vi "Main_UI.vi"() -> ()   [LabVIEW 2020, in "Airplane CLD1.lvlib"]
doc: "This is an Airplane Lavatory. This shows if the front and rear are occupied. The Steward's area controls the signals and Alarm."
uses:
  Airplane CLD1.lvlib
  Input_Cluster.ctl
panel:
  in  "Stop":bool
  out "Error out":errorcluster
  in  "Error in":errorcluster
  in  "Alarm Timer Limit":dbl=10.0
  out "Alarm Timer D":dbl
  out "Alarm Timer C":dbl
  out "Alarm Timer B":dbl
  out "Alarm Timer A":dbl
  out "Lavatory":string
  in  "Alarm Acknowledge":bool
  out "Alarm":bool
  in  "Seatbelt Sign ON":bool
  out "Lavatories \nOccupied\nRear":bool
  out "Lavatories \nOccupied\nFront":bool
  in  "Lavatory D Occupied":bool
  in  "Lavatory C Occupied":bool
  in  "Lavatory B Occupied":bool
  in  "Lavatory A Occupied":bool
  out "Return to Seat B":bool
  out "Occupied B":bool
  out "Return to Seat A":bool
  out "Occupied A":bool
  out "Return to Seat D":bool
  out "Occupied D":bool
  out "Return to Seat C":bool
  out "Occupied C":bool
  # "AIRPLANE LAVATORY SIGNS"
  # "FRONT"
  # "REAR"
  # "LAVATORY A"
  # "LAVATORY C"
  # "STEWARDS'S AREA"
  # "LAVATORY B"
  # "LAVATORY D"
  # "SIMULATION CONTROLS & INDICATORS"
  # "secs"
  # "secs"
  # "secs"
  # "secs"
  # "secs"
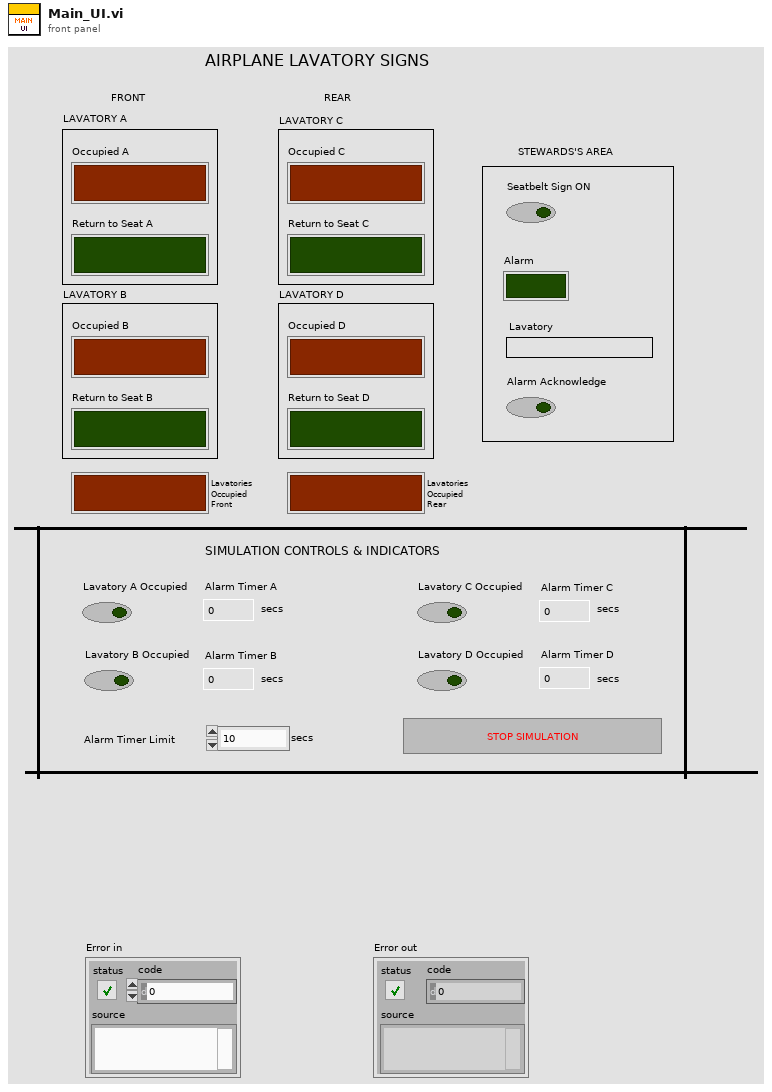
[diagram p1: front panel]
types:
  T1 = typedef "Airplane CLD1.lvlib/Input_Cluster.ctl" = cluster{"Occupied A":bool, "Occupied B":bool, "Occupied C ":bool, "Occupied D":bool, "Lavatories \nOccupied\nFront":bool, "Lavatories \nOccupied\nRear":bool, "Return":bool, "A Initial":dbl, "B Initial":dbl, "C Initial":dbl, "D Initial":dbl, "Alarm Timer A":dbl, "Alarm Timer B":dbl, "Alarm Timer C":dbl, "Alarm Timer D":dbl, "Alarm Timer Limit":dbl, "Lavatory":string, "Alarm":bool, "Alarm Acknowledge":bool}
  T2 = enum16{"Create Queue", "Enqueue element", "Enqueue N elements", "Dequeue", "Enstack 1 element", "Flush Queue", "Close Queue"}
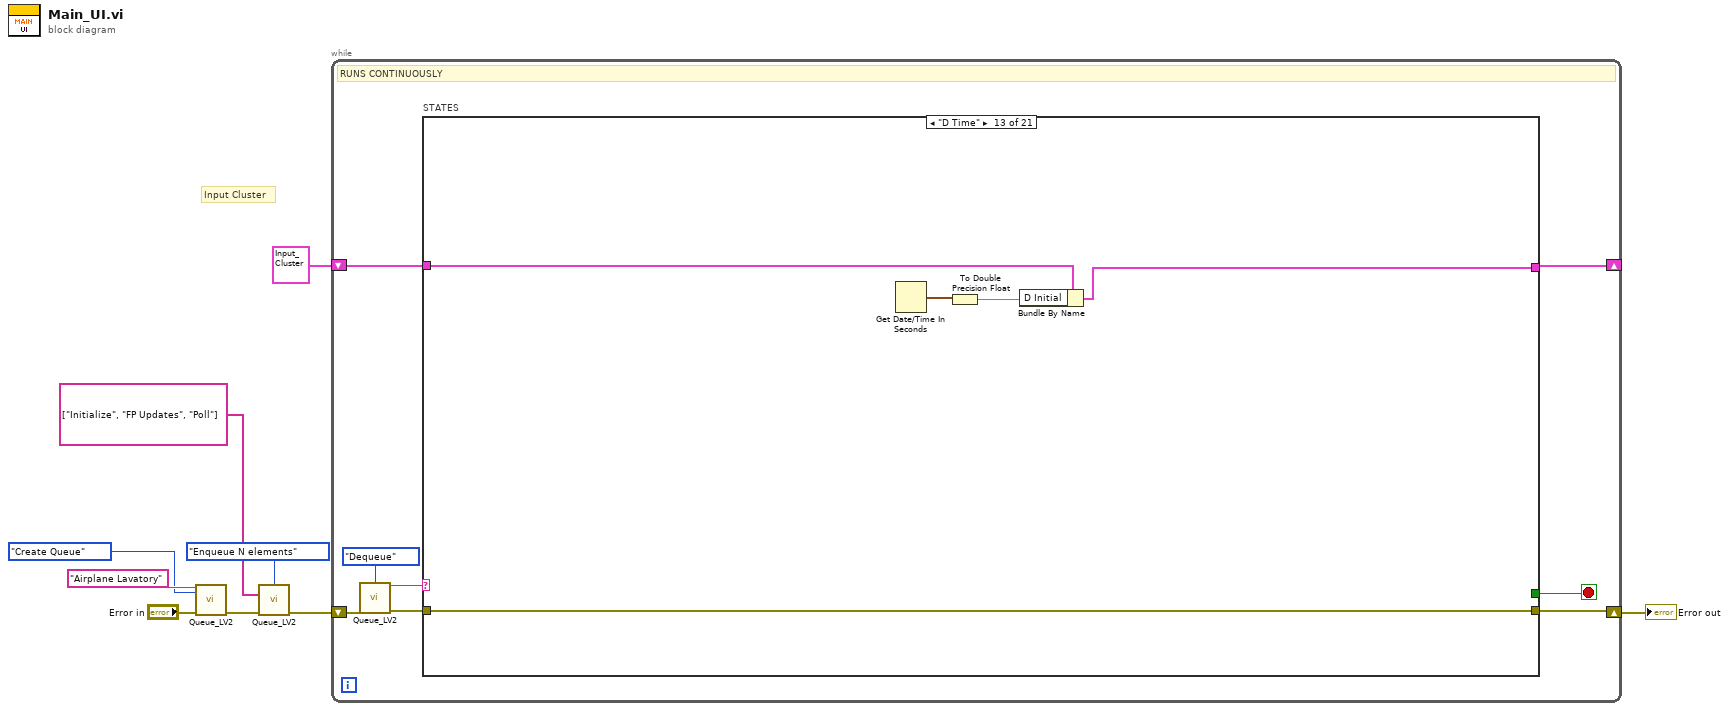
[diagram p0: block diagram]
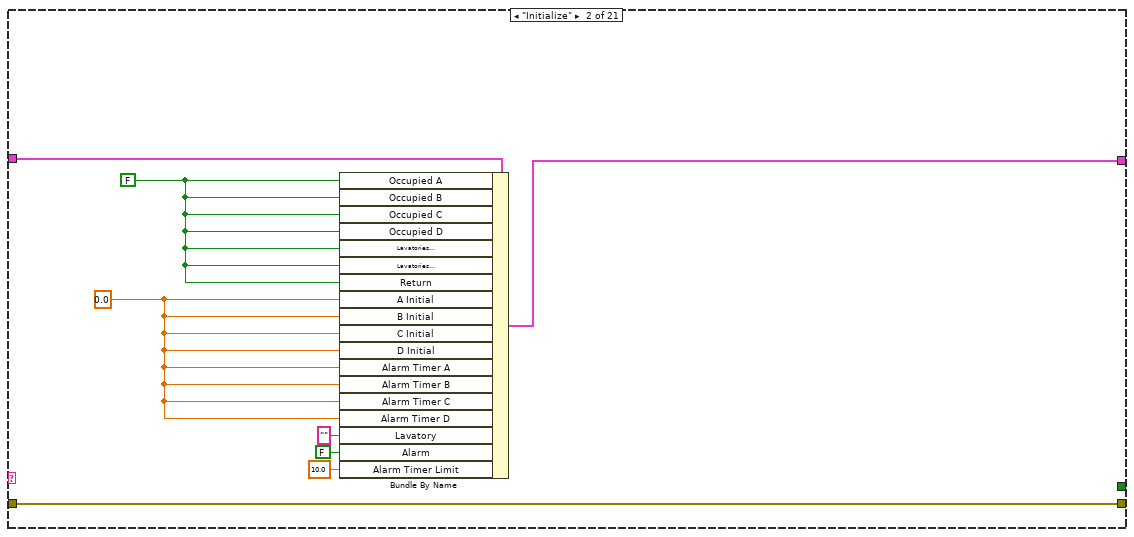
[diagram p3: hidden frame]
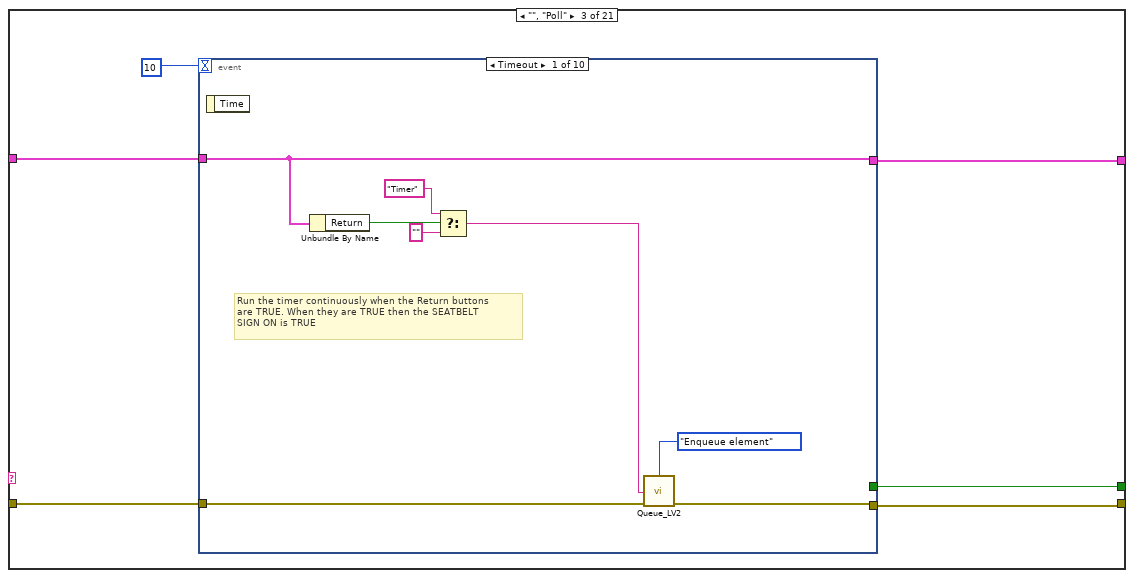
[diagram p4: hidden frame]
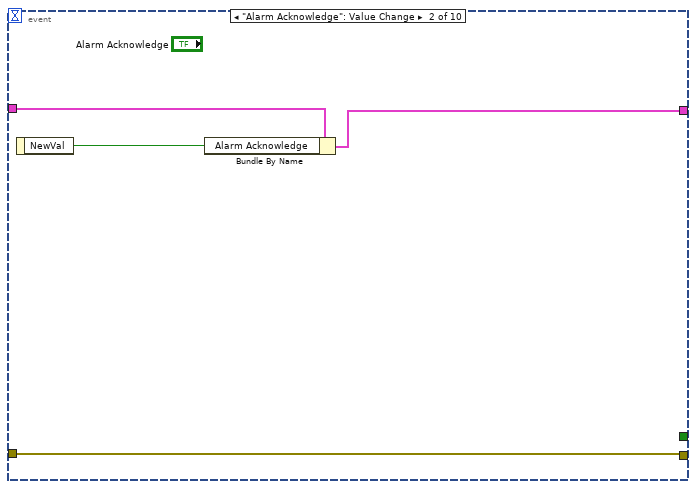
[diagram p5: hidden frame]
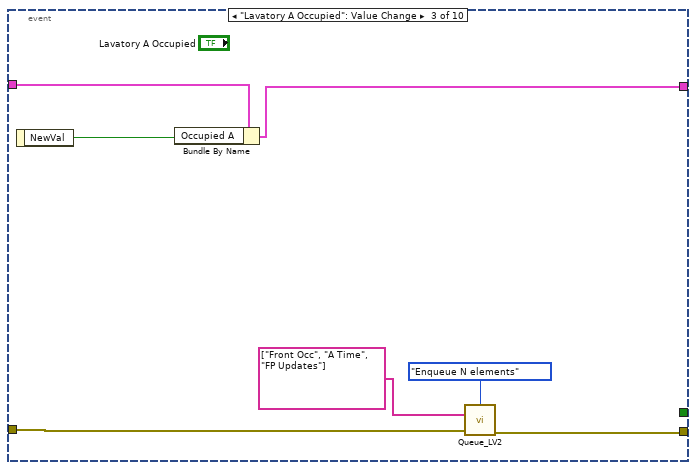
[diagram p6: hidden frame]
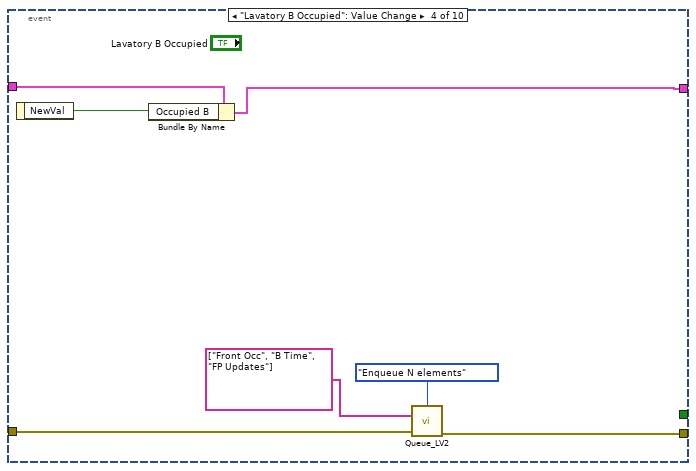
[diagram p7: hidden frame]
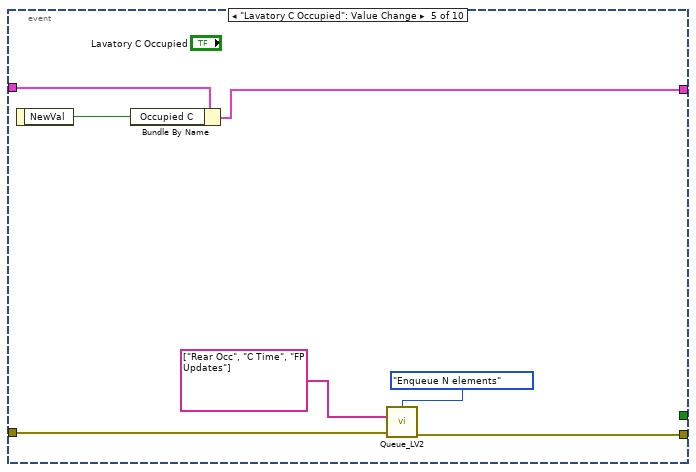
[diagram p8: hidden frame]
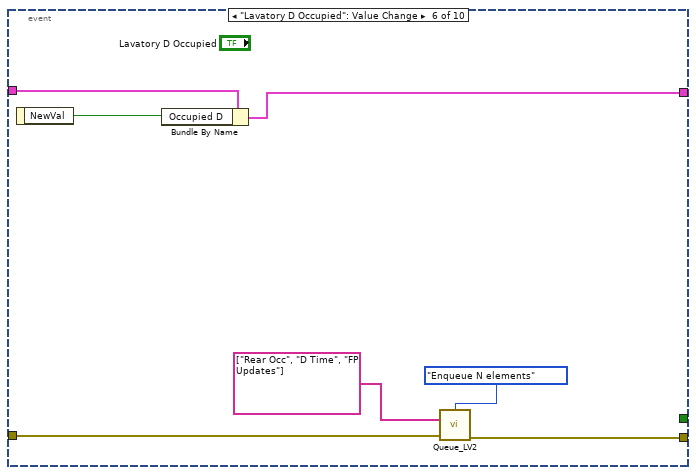
[diagram p9: hidden frame]
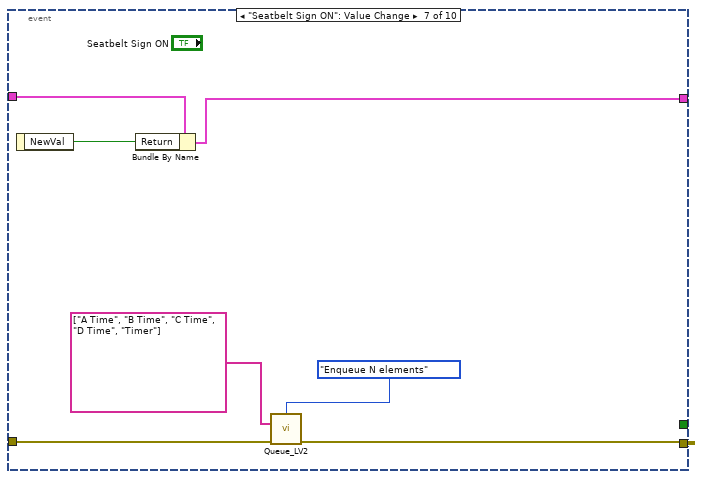
[diagram p10: hidden frame]
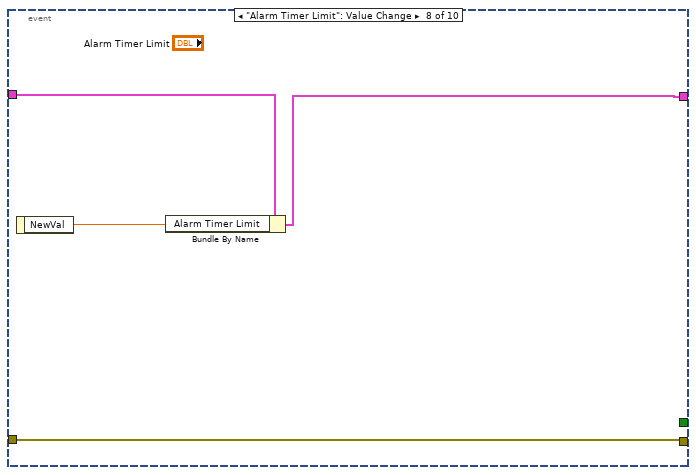
[diagram p11: hidden frame]
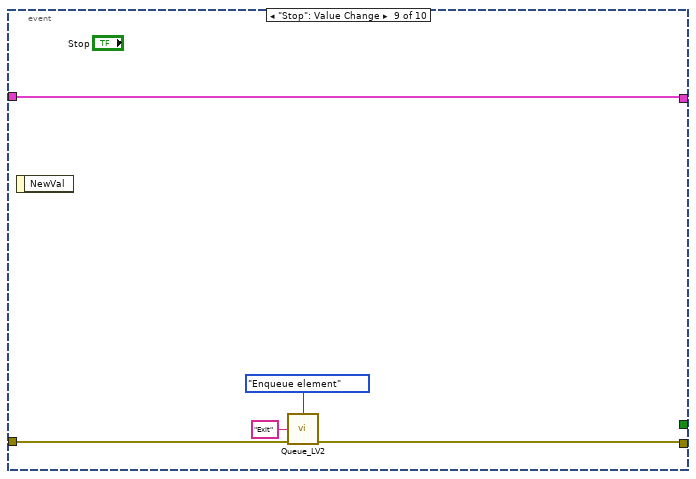
[diagram p12: hidden frame]
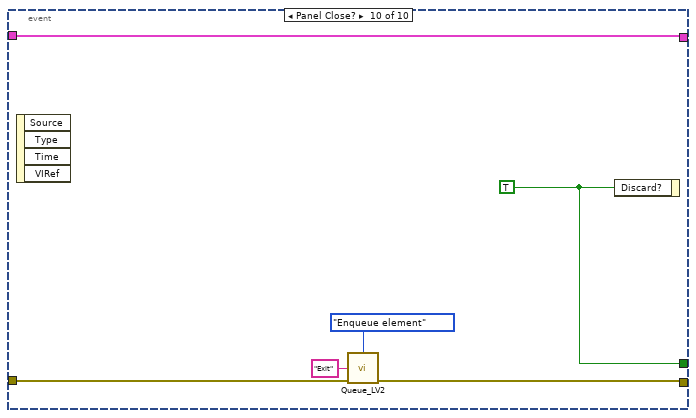
[diagram p13: hidden frame]
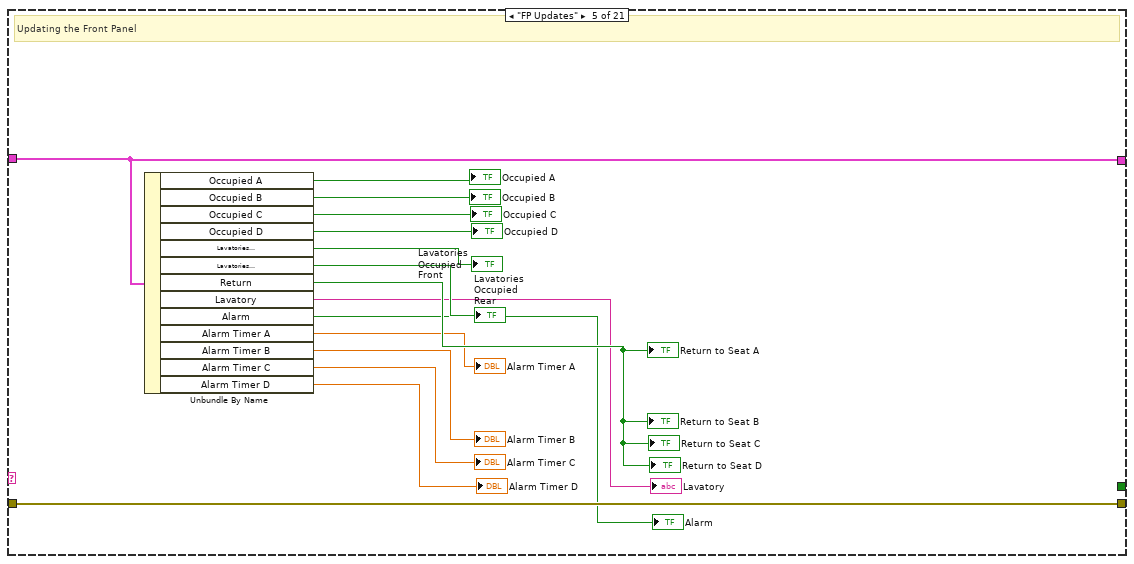
[diagram p15: hidden frame]
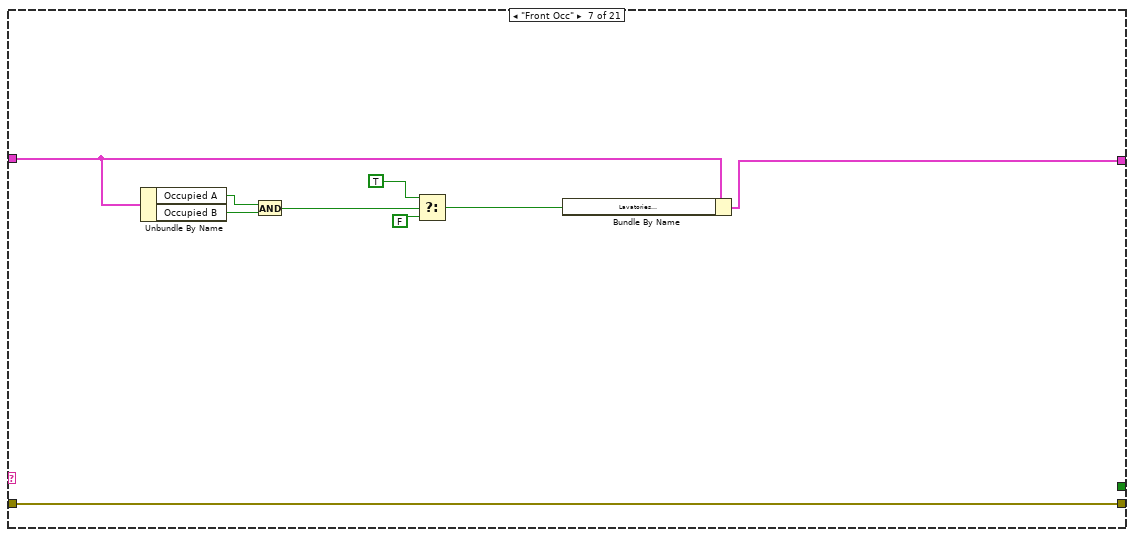
[diagram p17: hidden frame]
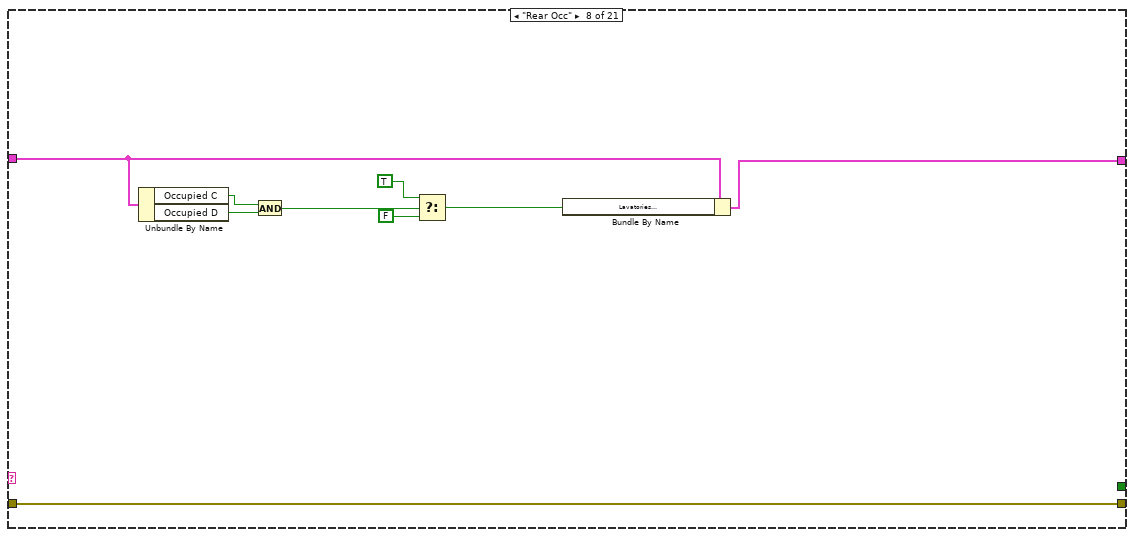
[diagram p18: hidden frame]
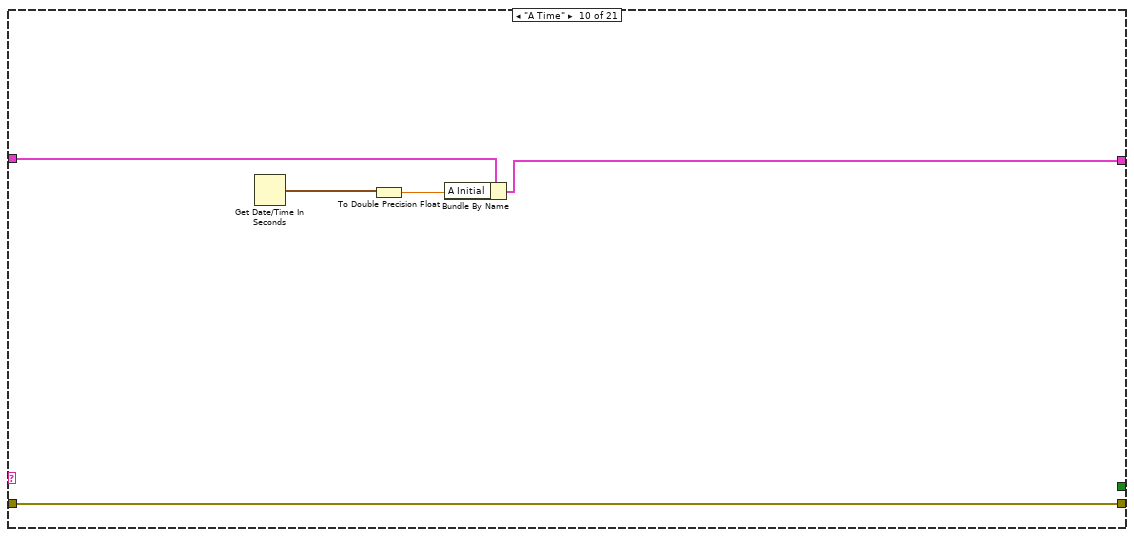
[diagram p20: hidden frame]
diagram:
  # "Input Cluster"
  n1 = call "Queue_LV2.vi"("name"="Airplane Lavatory", "Queue Operations"=T2."Create Queue", "error in"="Error in") -> ("error out"=w7:errorcluster)  [unwired: 11 in, 1 out]
  n2 = call "Queue_LV2.vi"("Queue Operations"=T2."Enqueue N elements", "States[]"=string[] ["Initialize", "FP Updates", "Poll"], "error in"=w7) -> ("error out"=w5:errorcluster)  [unwired: 11 in, 1 out]
  n3 = while {
    shift-right: [w13] -> w2
    shift-left: w5 -> [w17]
    shift-right: [w10] -> _
    shift-left: T1 {"Occupied A"=FALSE, "Occupied B"=FALSE, "Occupied C "=FALSE, "Occupied D"=FALSE, "Lavatories \nOccupied\nFront"=FALSE, "Lavatories \nOccupied\nRear"=FALSE, "Return"=FALSE, "A Initial"=0.0, "B Initial"=0.0, "C Initial"=0.0, "D Initial"=0.0, "Alarm Timer A"=0.0, "Alarm Timer B"=0.0, "Alarm Timer C"=0.0, "Alarm Timer D"=0.0, "Alarm Timer Limit"=0.0, "Lavatory"="", "Alarm"=FALSE, "Alarm Acknowledge"=FALSE} -> [w11]
    stop <- w12 stop-if-true
    # "RUNS CONTINUOUSLY"
    n4 = call "Queue_LV2.vi"("Queue Operations"=T2."Dequeue", "error in"=w17) -> ("DQ State"=w15:string, "error out"=w14:errorcluster)  [unwired: 12 in]
    n5 = case "STATES" shown="\"D Time\"" w15 {
      selector: w15 -> [_ _ _ _ _ _ _ _ _ _ _ _ _ _ _ _ _ _ w249 _ _]
      tunnel: w14 -> [w19 w27 w30 w96 w107 w113 w123 w132 w133 w135 w140 w145 w150 w155 w158 w190 w204 w245 w250 w251 w258]
      tunnel: [w19 w27 w29 w96 w107 w113 w123 w132 w133 w135 w140 w145 w150 w155 w159 w190 w200 w245 w250 w251 w254] -> w13
      tunnel: [_ _ w28 _ _ _ _ _ _ _ _ _ _ _ _ _ _ _ w248 _ TRUE ("true")] -> w12
      tunnel: w11 -> [w18 w26 w32 w97 w108 w114 w117 w124 w134 w139 w142 w147 w152 w156 w166 w191 w219 w246 w247 w252 w259]
      tunnel: [w18 w25 w31 w97 w108 w114 w116 w125 w134 w136 w141 w146 w151 w156 w165 w191 w217 w246 w247 w252 w259] -> w10
      frame "/****Initialize****/" {
        # "Splitter Case"
      }
      frame "Initialize" {
        w23 = 0.0
        w24 = FALSE ("Occupied A")
        n6 = Bundle By Name(cluster=w26, "Occupied A"=w24, "Occupied B"=w24, "Occupied C"=w24, "Occupied D"=w24, "Lavatories \nOccupied\nFront"=w24, "Lavatories \nOccupied\nRear"=w24, "Return"=w24, "A Initial"=w23, "B Initial"=w23, "C Initial"=w23, "D Initial"=w23, "Alarm Timer A"=w23, "Alarm Timer B"=w23, "Alarm Timer C"=w23, "Alarm Timer D"=w23, "Lavatory"="", "Alarm"=FALSE, "Alarm Timer Limit"=10.0) -> (w25:T1)
      }
      frame "", "Poll" {
        n7 = event shown="[0] Timeout" {
          selector: _ -> [_ _ _ _ _ _ _ _ _ _]
          dyn-events: _ -> [_ _ _ _ _ _ _ _ _ _]
          timeout: 10 -> [_ _ _ _ _ _ _ _ _ _]
          tunnel: w32 -> [w41 w45 w52 w59 w66 w73 w80 w84 w85 w94]
          tunnel: [w41 w44 w50 w58 w65 w72 w78 w82 w85 w94] -> w31
          tunnel: w30 -> [w35 w42 w47 w54 w61 w70 w77 w81 w89 w93]
          tunnel: [w34 w42 w46 w53 w60 w69 w76 w81 w88 w92] -> w29
          tunnel: [_ _ _ _ _ _ _ _ _ w95] -> w28
          event Timeout {
            # "Run the timer continuously when the Return buttons\nare TRUE. When they are TRUE then the SEATBELT\nSIGN ON is TRUE"
            n8 = event-data() -> ()  [unwired: 1 in, 1 out]
            n9 = Unbundle By Name(w41) -> ("Return"=w40:bool)
            n10 = Select(t="Timer", s=w40, f="") -> (s? t:f=w37:string)
            n11 = call "Queue_LV2.vi"("Queue Operations"=T2."Enqueue element", "State"=w37, "error in"=w35) -> ("error out"=w34:errorcluster)  [unwired: 11 in, 1 out]
          }
          event "Alarm Acknowledge": Value Change {
            n12 = event-data() -> ("NewVal"=w43:bool)  [unwired: 1 in]
            n13 = Bundle By Name(cluster=w45, "Alarm Acknowledge"=w43) -> (w44:T1)
          }
          event "Lavatory A Occupied": Value Change {
            n14 = event-data() -> ("NewVal"=w51:bool)  [unwired: 1 in]
            n15 = Bundle By Name(cluster=w52, "Occupied A"=w51) -> (w50:T1)
            n16 = call "Queue_LV2.vi"("Queue Operations"=T2."Enqueue N elements", "States[]"=string[] ["Front Occ", "A Time", "FP Updates"], "error in"=w47) -> ("error out"=w46:errorcluster)  [unwired: 11 in, 1 out]
          }
          event "Lavatory B Occupied": Value Change {
            n17 = event-data() -> ("NewVal"=w57:bool)  [unwired: 1 in]
            n18 = Bundle By Name(cluster=w59, "Occupied B"=w57) -> (w58:T1)
            n19 = call "Queue_LV2.vi"("Queue Operations"=T2."Enqueue N elements", "States[]"=string[] ["Front Occ", "B Time", "FP Updates"], "error in"=w54) -> ("error out"=w53:errorcluster)  [unwired: 11 in, 1 out]
          }
          event "Lavatory C Occupied": Value Change {
            n20 = event-data() -> ("NewVal"=w64:bool)  [unwired: 1 in]
            n21 = Bundle By Name(cluster=w66, "Occupied C"=w64) -> (w65:T1)
            n22 = call "Queue_LV2.vi"("Queue Operations"=T2."Enqueue N elements", "States[]"=string[] ["Rear Occ", "C Time", "FP Updates"], "error in"=w61) -> ("error out"=w60:errorcluster)  [unwired: 11 in, 1 out]
          }
          event "Lavatory D Occupied": Value Change {
            n23 = event-data() -> ("NewVal"=w71:bool)  [unwired: 1 in]
            n24 = Bundle By Name(cluster=w73, "Occupied D"=w71) -> (w72:T1)
            n25 = call "Queue_LV2.vi"("Queue Operations"=T2."Enqueue N elements", "States[]"=string[] ["Rear Occ", "D Time", "FP Updates"], "error in"=w70) -> ("error out"=w69:errorcluster)  [unwired: 11 in, 1 out]
          }
          event "Seatbelt Sign ON": Value Change {
            n26 = event-data() -> ("NewVal"=w79:bool)  [unwired: 1 in]
            n27 = Bundle By Name(cluster=w80, "Return"=w79) -> (w78:T1)
            n28 = call "Queue_LV2.vi"("Queue Operations"=T2."Enqueue N elements", "States[]"=string[] ["A Time", "B Time", "C Time", "D Time", "Timer"], "error in"=w77) -> ("error out"=w76:errorcluster)  [unwired: 11 in, 1 out]
          }
          event "Alarm Timer Limit": Value Change {
            n29 = event-data() -> ("NewVal"=w83:dbl)  [unwired: 1 in]
            n30 = Bundle By Name(cluster=w84, "Alarm Timer Limit"=w83) -> (w82:T1)
          }
          event "Stop": Value Change {
            n31 = event-data() -> ()  [unwired: 1 in, 1 out]
            n32 = call "Queue_LV2.vi"("Queue Operations"=T2."Enqueue element", "State"="Exit", "error in"=w89) -> ("error out"=w88:errorcluster)  [unwired: 11 in, 1 out]
          }
          event Panel Close? {
            w95 = TRUE ("Discard?")
            n33 = event-data() -> ()  [unwired: 1 in, 4 out]
            n34 = call "Queue_LV2.vi"("Queue Operations"=T2."Enqueue element", "State"="Exit", "error in"=w93) -> ("error out"=w92:errorcluster)  [unwired: 11 in, 1 out]
            n35 = event-data("Discard?"=w95) -> ()  [unwired: 1 in, 1 out]
          }
        }
      }
      frame "/****FP Updates****/" {
        # "Splitter Case"
      }
      frame "FP Updates" {
        # "Updating the Front Panel"
        n36 = Unbundle By Name(w108) -> ("Occupied A"=→"Occupied A":bool, "Occupied B"=→"Occupied B":bool, "Occupied C"=→"Occupied C":bool, "Occupied D"=→"Occupied D":bool, "Lavatories \nOccupied\nFront"=→"Lavatories \nOccupied\nFront":bool, "Lavatories \nOccupied\nRear"=→"Lavatories \nOccupied\nRear":bool, "Return"=→"Return to Seat C" →"Return to Seat D" →"Return to Seat A" →"Return to Seat B":bool, "Lavatory"=→"Lavatory":string, "Alarm"=→"Alarm":bool, "Alarm Timer A"=→"Alarm Timer A":dbl, "Alarm Timer B"=→"Alarm Timer B":dbl, "Alarm Timer C"=→"Alarm Timer C":dbl, "Alarm Timer D"=→"Alarm Timer D":dbl)
      }
      frame "/****Front and Rear Update****/" {
        # "Splitter Case"
      }
      frame "Front Occ" {
        n37 = Unbundle By Name(w117) -> ("Occupied A"=w122:bool, "Occupied B"=w121:bool)
        n38 = And(x=w122, y=w121) -> (x .and. y?=w120:bool)
        n39 = Select(t=TRUE, s=w120, f=FALSE) -> (s? t:f=w115:bool)
        n40 = Bundle By Name(cluster=w117, "Lavatories \nOccupied\nFront"=w115) -> (w116:T1)
      }
      frame "Rear Occ" {
        n41 = Unbundle By Name(w124) -> ("Occupied C"=w131:bool, "Occupied D"=w130:bool)
        n42 = And(x=w131, y=w130) -> (x .and. y?=w129:bool)
        n43 = Select(t=TRUE, s=w129, f=FALSE) -> (s? t:f=w126:bool)
        n44 = Bundle By Name(cluster=w124, "Lavatories \nOccupied\nRear"=w126) -> (w125:T1)
      }
      frame "/****Time of Lavatory press****/" {
        # "Splitter Case"
      }
      frame "A Time" {
        n45 = Get Date/Time In Seconds() -> (seconds since 1Jan1904=w138:timestamp)
        n46 = To Double Precision Float(number=w138) -> (double precision float=w137:dbl)
        n47 = Bundle By Name(cluster=w139, "A Initial"=w137) -> (w136:T1)
      }
      frame "B Time" {
        n48 = Get Date/Time In Seconds() -> (seconds since 1Jan1904=w143:timestamp)
        n49 = To Double Precision Float(number=w143) -> (double precision float=w144:dbl)
        n50 = Bundle By Name(cluster=w142, "B Initial"=w144) -> (w141:T1)
      }
      frame "C Time" {
        n51 = Get Date/Time In Seconds() -> (seconds since 1Jan1904=w148:timestamp)
        n52 = To Double Precision Float(number=w148) -> (double precision float=w149:dbl)
        n53 = Bundle By Name(cluster=w147, "C Initial"=w149) -> (w146:T1)
      }
      frame "D Time" {
        n54 = Get Date/Time In Seconds() -> (seconds since 1Jan1904=w153:timestamp)
        n55 = To Double Precision Float(number=w153) -> (double precision float=w154:dbl)
        n56 = Bundle By Name(cluster=w152, "D Initial"=w154) -> (w151:T1)
      }
      frame "/****Timer****/" {
        # "Splitter Case"
      }
      frame "Timer" {
        # "Current Time"
        n57 = Unbundle By Name(w166) -> ("A Initial"=w187:dbl, "B Initial"=w186:dbl, "C Initial"=w185:dbl, "D Initial"=w184:dbl, "Occupied A"=w183:bool, "Occupied B"=w180:bool, "Occupied C"=w179:bool, "Occupied D"=w178:bool, "Return"=w177:bool)
        n58 = Get Date/Time In Seconds() -> (seconds since 1Jan1904=w189:timestamp)
        n59 = To Double Precision Float(number=w189) -> (double precision float=w188:dbl)
        n60 = Subtract(x=w188, y=w187) -> (x-y=w181:dbl)
        n61 = Subtract(x=w188, y=w186) -> (x-y=w174:dbl)
        n62 = Subtract(x=w188, y=w185) -> (x-y=w171:dbl)
        n63 = Subtract(x=w188, y=w184) -> (x-y=w169:dbl)
        n64 = And(x=w183, y=w177) -> (x .and. y?=w182:bool)
        n65 = And(x=w180, y=w177) -> (x .and. y?=w175:bool)
        n66 = And(x=w178, y=w177) -> (x .and. y?=w168:bool)
        n67 = And(x=w179, y=w177) -> (x .and. y?=w172:bool)
        n68 = Select(t=w169, s=w168, f=0.0) -> (s? t:f=w161:dbl)
        n69 = Select(t=w174, s=w175, f=0.0) -> (s? t:f=w163:dbl)
        n70 = Select(t=w171, s=w172, f=0.0) -> (s? t:f=w162:dbl)
        n71 = Select(t=w181, s=w182, f=0.0) -> (s? t:f=w164:dbl)
        n72 = Bundle By Name(cluster=w166, "Alarm Timer A"=w164, "Alarm Timer B"=w163, "Alarm Timer C"=w162, "Alarm Timer D"=w161) -> (w165:T1)
        n73 = call "Queue_LV2.vi"("Queue Operations"=T2."Enqueue N elements", "States[]"=string[] ["Alarm Limit", "FP Updates"], "error in"=w158) -> ("error out"=w159:errorcluster)  [unwired: 11 in, 1 out]
      }
      frame "/****Alarm Limit Check****/" {
        # "Splitter Case"
      }
      frame "Alarm Limit" {
        w213 = "" ("f")
        n74 = Unbundle By Name(w219) -> ("Alarm Timer A"=w224:dbl, "Alarm Timer B"=w223:dbl, "Alarm Timer C"=w222:dbl, "Alarm Timer D"=w221:dbl, "Alarm Timer Limit"=w220:dbl, "Alarm Acknowledge"=w195:bool)
        n75 = Greater?(x=w224, y=w220) -> (0:w206:bool)
        n76 = Greater?(x=w223, y=w220) -> (0:w199:bool)
        n77 = Greater?(x=w222, y=w220) -> (0:w197:bool)
        n78 = Greater?(x=w221, y=w220) -> (0:w194:bool)
        n79 = And(x=w206, y=w195) -> (x .and. y?=w205:bool)
        n80 = case shown="False" w205 {
          tunnel: w204 -> [w240 w244]
          tunnel: [w240 w241] -> w203
          frame False {
          }
          frame True {
            # "Reset"
            n81 = call "Queue_LV2.vi"("Queue Operations"=T2."Enstack 1 element", "State"="A Time", "error in"=w244) -> ("error out"=w241:errorcluster)  [unwired: 11 in, 1 out]
          }
        }
        n82 = And(x=w195, y=w199) -> (x .and. y?=w198:bool)
        n83 = case shown="True" w198 {
          tunnel: w203 -> [w235 w239]
          tunnel: [w235 w236] -> w202
          frame False {
          }
          frame True {
            # "Reset"
            n84 = call "Queue_LV2.vi"("Queue Operations"=T2."Enstack 1 element", "State"="B Time", "error in"=w239) -> ("error out"=w236:errorcluster)  [unwired: 11 in, 1 out]
          }
        }
        n85 = And(x=w195, y=w197) -> (x .and. y?=w196:bool)
        n86 = Compound Arithmetic op=OR(w206, w199, w197, w194) -> (w218:bool)
        n87 = Select(t="A", s=w206, f=w213) -> (s? t:f=w211:string)
        n88 = Select(t="B", s=w199, f=w213) -> (s? t:f=w210:string)
        n89 = Select(t="C", s=w197, f=w213) -> (s? t:f=w209:string)
        n90 = Select(t="D", s=w194, f=w213) -> (s? t:f=w208:string)
        n91 = Concatenate Strings(w211, w210, w209, w208) -> (w207:string)
        n92 = case shown="True" w196 {
          tunnel: w202 -> [w230 w234]
          tunnel: [w230 w231] -> w201
          frame False {
          }
          frame True {
            # "Reset"
            n93 = call "Queue_LV2.vi"("Queue Operations"=T2."Enstack 1 element", "State"="C Time", "error in"=w234) -> ("error out"=w231:errorcluster)  [unwired: 11 in, 1 out]
          }
        }
        n94 = And(x=w195, y=w194) -> (x .and. y?=w193:bool)
        n95 = case shown="True" w193 {
          tunnel: w201 -> [w225 w229]
          tunnel: [w225 w226] -> w200
          frame False {
          }
          frame True {
            # "Reset"
            n96 = call "Queue_LV2.vi"("Queue Operations"=T2."Enstack 1 element", "State"="D Time", "error in"=w229) -> ("error out"=w226:errorcluster)  [unwired: 11 in, 1 out]
          }
        }
        n97 = Bundle By Name(cluster=w219, "Alarm"=w218, "Lavatory"=w207, "Alarm Acknowledge"=FALSE) -> (w217:T1)
      }
      frame "/****Default****/" {
        # "Splitter Case"
      }
      frame Default {
        n98 = One Button Dialog(message=w249) -> (true=w248:bool)  [unwired: 1 in]
      }
      frame "/****Exit****/" {
        # "Splitter Case"
      }
      frame "Exit" {
        n99 = call "Queue_LV2.vi"("Queue Operations"=T2."Flush Queue", "error in"=w258) -> ("error out"=w256:errorcluster)  [unwired: 12 in, 1 out]
        n100 = call "Queue_LV2.vi"("Queue Operations"=T2."Close Queue", "error in"=w256) -> ("error out"=w254:errorcluster)  [unwired: 12 in, 1 out]
      }
    }
  }
  "Error out" <- w2
